vi "Get Software Version.vi"(8 "error in (no error)":errorcluster, 11 "Ethernet in":refnum<class "ENET_BS1200.lvclass">) -> (0 "error out":errorcluster, 2 "Version":string, 3 "Ethernet out":refnum<class "ENET_BS1200.lvclass">)   [LabVIEW 2021, in "BS120x Driver.lvlib" / "ENET_BS1200.lvclass"]
doc: "Retrieve Battery Simulator 1200 firmware version.\n(c) 2019 Bloomy Controls, Inc. All rights reserved."
uses:
  ENET_BS1200.lvclass
  <vilib>/nisyscfg/Close (System).vi
  <resource>/objmgr/nisysapi.rc
  <vilib>/nisyscfg/nisyscfg.lvlib
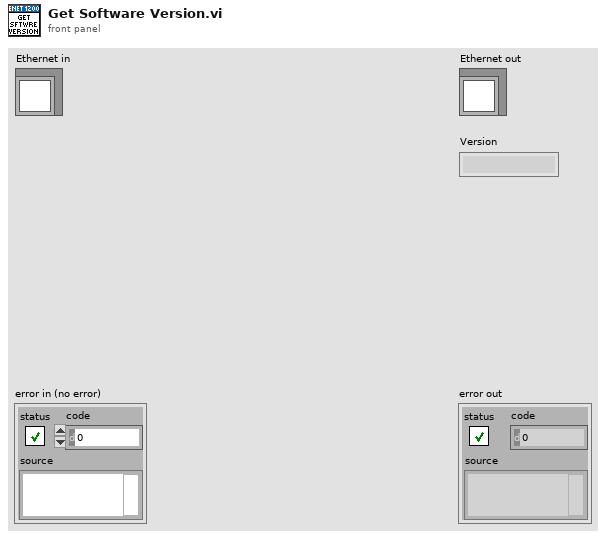
[diagram p1: front panel]
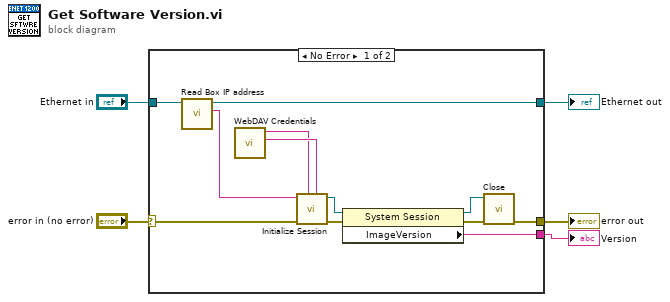
[diagram p0: block diagram]
diagram:
  n1 = case shown="No Error" "error in (no error)" {
    selector: "error in (no error)" -> [w17 w19]
    tunnel: [w9 w19] -> w4
    tunnel: [w7 w18] -> w2
    tunnel: "Ethernet in" -> [w8 w18]
    tunnel: [w10 _] -> w1
    frame No Error {
      n2 = call-dynamic "Read Box IP address.vi"("ENET_BS120x in"=w8) -> ("Box IP address"=w6:string, "ENET_BS120x out"=w7:refnum<class "ENET_BS1200.lvclass">)  [unwired: 8 in, 1 out]
      n3 = call "WebDAV Credentials.vi"() -> ("Password"=w12:string, "Username"=w11:string)  [unwired: 10 in]
      n4 = call <vilib>:"Initialize Session.vi"("Password"=w12, "User Name"=w11, "error in (no error)"=w17, "Target (localhost)"=w6) -> ("error out"=w15:errorcluster, "Session out"=w16:refnum<k21>)  [unwired: 6 in]
      n5 = property class="System Session"(reference=w16, error in=w15) -> (reference out=w13:refnum<k21>, error out=w14:errorcluster, "ImageVersion"=w10:string)
      n6 = call-poly <vilib>:"Close.vi"("error in (no error)"=w14, "Session in"=w13) -> ("error out"=w9:errorcluster)  [unwired: 9 in]
    }
    frame Error {
    }
  }
  "error out" <- w4
  "Ethernet out" <- w2
  "Version" <- w1
